vi "rostopic_write_test.vi"() -> ()   [LabVIEW 2012]
uses:
  <userlib>/rosforlv/ROS/Code/Console/Servers/ServerSubs/TopicDef.ctl
  <userlib>/rosforlv/ROS/Code/SubVIs/_ROSDirection.ctl
  <userlib>/rosforlv/ROS/parsing/std_msgs/subs/parse_string_scalar.vi
  <userlib>/rosforlv/ROS/MessageBuilding/std_msgs/subs/stringScalar.vi
panel:
  in  "write msg":string="what now?"
  in  "stop read":bool
  in  "stop write":bool
  out "Read Msg":string
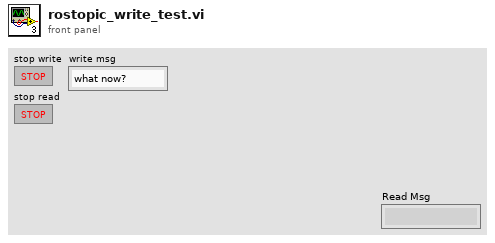
[diagram p1: front panel]
types:
  T1 = typedef "TopicDef.ctl" = cluster{"Topic":string, "Type":string, "Action":T2, "Update (ms)":u16, "write queue":u16}
  T2 = typedef "_ROSDirection.ctl" = enum16{"Node", "Publisher", "Subscriber", "Service Client"}
  T3 = typedef "_ROSControl.ctl" = cluster{"topic port":u16, "Node":string, "topic":string, "type":string, "node port":u32, "error ":errorcluster, "Direction":T2, "APIs":string[], "Update (ms)":u16, "write queue":u16}
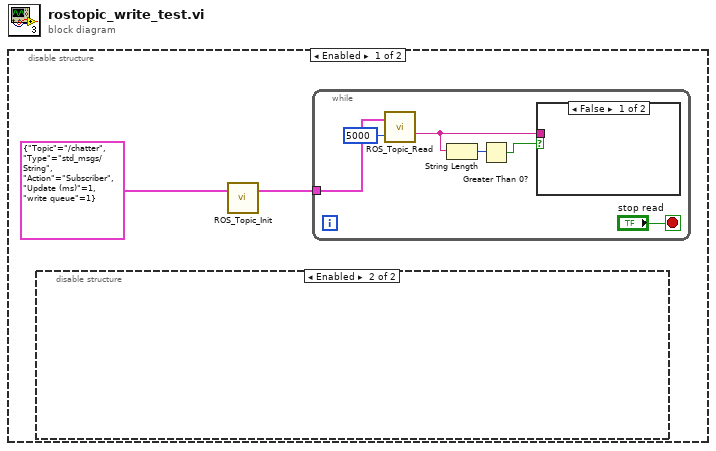
[diagram p0: block diagram]
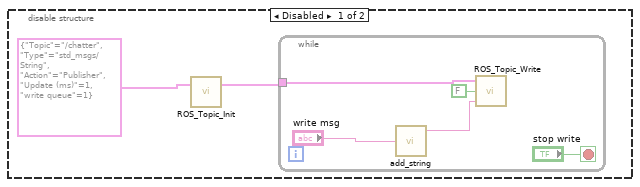
[diagram p2: hidden frame]
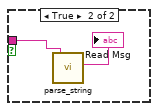
[diagram p3: hidden frame]
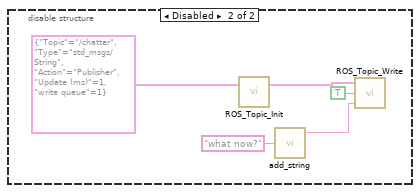
[diagram p4: hidden frame]
diagram:
  n1 = disable-structure shown="Enabled" {
    frame Enabled {
      n2 = disable-structure shown="Enabled" {
        frame Disabled {
          n3 = call <userlib>:"ROS_Topic_Init.vi"("Definitions"=T1 {"Topic"="/chatter", "Type"="std_msgs/String", "Action"=enum."Publisher", "Update (ms)"=1, "write queue"=1}) -> ("ROS out"=w3:T3)  [unwired: 2 in]
          n4 = while {
            tunnel: w3 -> [w5]
            stop <- "stop write" stop-if-true
            n5 = call-poly <userlib>:"add_string.vi"("String"="write msg") -> ("msg out"=w8:string)  [unwired: 4 in]
            n6 = call <userlib>:"ROS_Topic_Write.vi"("Msg in"=w8, "Continuous?"=FALSE, "ROS in"=w5) -> ()  [unwired: 1 in, 1 out]
          }
        }
        frame Enabled {
        }
      }
      n7 = call <userlib>:"ROS_Topic_Init.vi"("Definitions"=T1 {"Topic"="/chatter", "Type"="std_msgs/String", "Action"=enum."Subscriber", "Update (ms)"=1, "write queue"=1}) -> ("ROS out"=w1:T3)  [unwired: 2 in]
      n8 = while {
        tunnel: w1 -> [w15]
        stop <- "stop read" stop-if-true
        n9 = call <userlib>:"ROS_Topic_Read.vi"("Timeout (ms)"=5000, "ROS in"=w15) -> ("Reply"=w13:string)  [unwired: 1 out]
        n10 = String Length(string=w13) -> (length=w12:i32)
        n11 = Greater Than 0?(x=w12) -> (x > 0?=w11:bool)
        n12 = case shown="False" w11 {
          tunnel: w13 -> [_ w17]
          frame False {
          }
          frame True {
            n13 = call-poly <userlib>:"parse_string.vi"("type"=w17, "msg in"=w17) -> ("string"=→"Read Msg":string)  [unwired: 3 in, 2 out]
          }
        }
      }
    }
    frame Disabled {
      n14 = call <userlib>:"ROS_Topic_Init.vi"("Definitions"=T1 {"Topic"="/chatter", "Type"="std_msgs/String", "Action"=enum."Publisher", "Update (ms)"=1, "write queue"=1}) -> ("ROS out"=w21:T3)  [unwired: 2 in]
      n15 = call-poly <userlib>:"add_string.vi"("String"="what now?") -> ("msg out"=w19:string)  [unwired: 4 in]
      n16 = call <userlib>:"ROS_Topic_Write.vi"("Msg in"=w19, "Continuous?"=TRUE, "ROS in"=w21) -> ()  [unwired: 1 in, 1 out]
    }
  }
